vi "_DP2TDMData.vi"(6 "chunk size":u32=10000000, 8 "error in (no error)":errorcluster, 10 "DataPlugin Object in":refnum<k20>, 11 "TDM Object in":refnum<k20>) -> (0 "error out":errorcluster, 2 "DataPlugin object out":refnum<k20>, 3 "TDM Object out":refnum<k20>)   [LabVIEW 2017]
doc: "Transfers data from the TDM storage to the TDMS file in chunks of a size specified in samples until all samples have been transferred."
uses:
  <vilib>/Utility/tdmsutil.llb/TDM2TDMSDatatypes.ctl
  <vilib>/Platform/storage/lvStorage.llb/_saveStringChannel.vi
  <vilib>/Platform/storage/lvStorage.llb/_saveInt16Channel.vi
  <vilib>/Platform/storage/lvStorage.llb/_saveFloat32Channel.vi
  <vilib>/Platform/storage/lvStorage.llb/_saveUInt8Channel.vi
  <vilib>/Platform/storage/lvStorage.llb/_saveInt32Channel.vi
  <vilib>/Platform/storage/lvStorage.llb/_saveFloat64Channel.vi
  <vilib>/Platform/storage/lvStorage.llb/_saveDateTimeChannel.vi
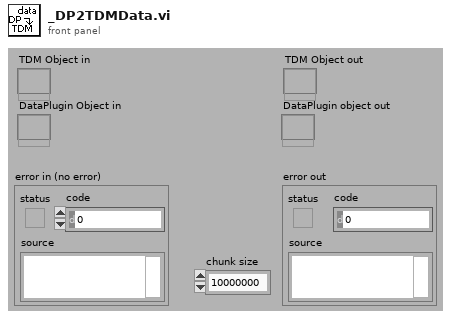
[diagram p1: front panel]
types:
  T1 = typedef "TDM2TDMSDatatypes.ctl" = enum16{"DT_UNKNOWN", "DT_STRING", "DT_SHORT", "DT_FLOAT", "DT_BOOLEAN", "DT_BYTE", "DT_LONG", "DT_DOUBLE", "DT_LONGLONG", "DT_ID", "DT_DATE", "DT_BYTESTR", "DT_BLOB", "DT_COMPLEX", "DT_DCOMPLEX", "DT_ENUM"}
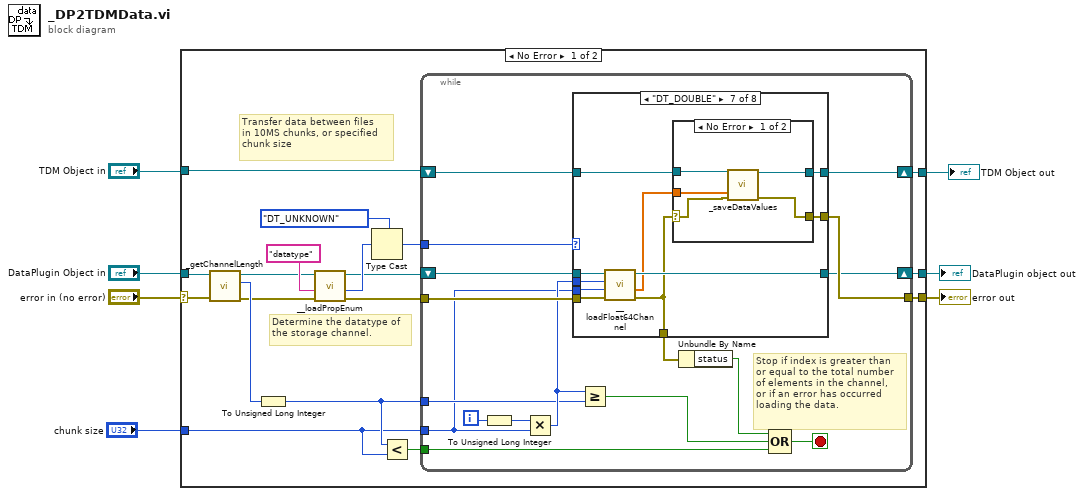
[diagram p0: block diagram]
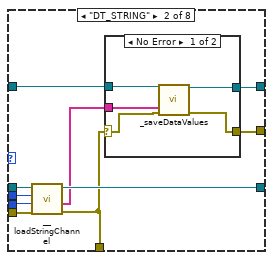
[diagram p3: hidden frame]
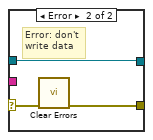
[diagram p4: hidden frame]
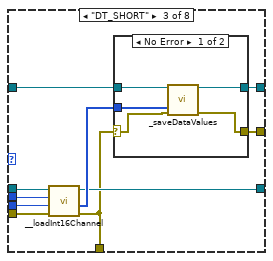
[diagram p5: hidden frame]
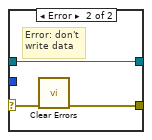
[diagram p6: hidden frame]
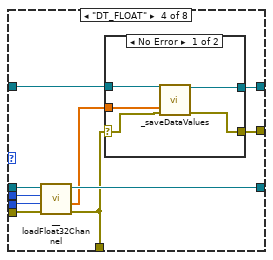
[diagram p7: hidden frame]
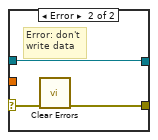
[diagram p8: hidden frame]
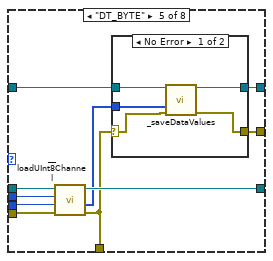
[diagram p9: hidden frame]
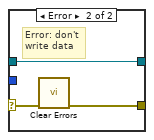
[diagram p10: hidden frame]
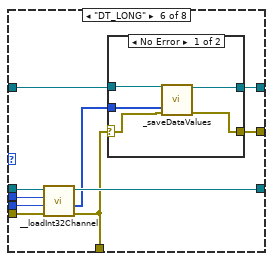
[diagram p11: hidden frame]
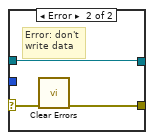
[diagram p12: hidden frame]
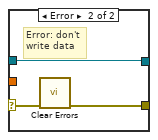
[diagram p13: hidden frame]
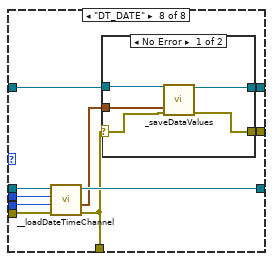
[diagram p14: hidden frame]
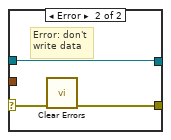
[diagram p15: hidden frame]
diagram:
  n1 = case shown="No Error" "error in (no error)" {
    selector: "error in (no error)" -> [w20 w172]
    tunnel: [w24 w174] -> w1
    tunnel: "DataPlugin Object in" -> [w21 w173]
    tunnel: "TDM Object in" -> [w23 w174]
    tunnel: [w22 w173] -> w2
    tunnel: [w25 w172] -> w7
    tunnel: "chunk size" -> [w9 _]
    frame No Error {
      # "Determine the datatype of\nthe storage channel."
      # "Transfer data between files\nin 10MS chunks, or specified\nchunk size"
      n2 = call <vilib>:"_getChannelLength.vi"("error in (no error)"=w20, "channel refnum in"=w21) -> ("error out"=w14:errorcluster, "channel length"=w19:i32, "channel refnum out"=w15:refnum<k20>)  [unwired: 3 in]
      n3 = To Unsigned Long Integer(number=w19) -> (unsigned 32bit integer=w10:u32)
      n4 = call <vilib>:"__loadPropEnum.vi"("error in (no error)"=w14, "Property name"="datatype", "storage refnum"=w15) -> ("error out"=w12:errorcluster, "Value"=w16:u16, "dup storage refnum"=w13:refnum<k20>)  [unwired: 5 in, 1 out]
      n5 = Type Cast(type=TDM2TDMSDatatypes."DT_UNKNOWN" ("Data type"), x=w16) -> (*(type *) &x=w11:T1)
      n6 = Less?(x=w10, y=w9) -> (x < y?=w8:bool)
      n7 = while {
        shift-right: [w42] -> w24
        shift-left: w23 -> [w40]
        shift-right: [w31] -> w22
        shift-left: w13 -> [w34]
        tunnel: [w39] -> w25
        tunnel: w10 -> [w28]
        tunnel: w9 -> [w27]
        tunnel: w12 -> [w35]
        tunnel: w11 -> [w36]
        tunnel: w8 -> [w26]
        i -> [w38]
        stop <- w41 stop-if-true
        # "Stop if index is greater than\nor equal to the total number\nof elements in the channel,\nor if an error has occurred\nloading the data."
        n8 = To Unsigned Long Integer(number=w38) -> (unsigned 32bit integer=w37:u32)
        n9 = Multiply(x=w37, y=w27) -> (x*y=w32:u32)
        n10 = case shown="\"DT_DOUBLE\"" w36 {
          tunnel: [w45 w50 w64 w86 w104 w121 w140 w157] -> w42
          tunnel: w40 -> [w45 w46 w73 w82 w103 w120 w138 w156]
          tunnel: [w44 w49 w66 w85 w100 w122 w139 w158] -> w39
          tunnel: w35 -> [w44 w54 w71 w90 w108 w126 w144 w162]
          tunnel: w34 -> [w43 w55 w72 w91 w109 w127 w145 w163]
          tunnel: w32 -> [_ w53 w70 w89 w107 w124 w143 w161]
          tunnel: w27 -> [_ w52 w69 w88 w106 w123 w142 w160]
          tunnel: [w43 w51 w67 w87 w105 w125 w141 w159] -> w31
          tunnel: [w44 w48 w65 w84 w102 w118 w136 w154] -> w30
          frame "DT_UNKNOWN", Default {
          }
          frame "DT_STRING" {
            n11 = call <vilib>:"__loadStringChannel.vi"("error in (no error)"=w54, "Count"=w52, "Index"=w53, "Data object in"=w55) -> ("error out"=w48:errorcluster, "Values"=w47:string[], "Data object out"=w51:refnum<k20>)  [unwired: 1 out]
            n12 = case shown="No Error" w48 {
              tunnel: [w60 w62] -> w49
              selector: w48 -> [w59 w63]
              tunnel: [w58 w61] -> w50
              tunnel: w47 -> [w57 _]
              tunnel: w46 -> [w56 w61]
              frame No Error {
                n13 = call-poly <vilib>:"_saveDataValues.vi"("Data object in"=w56, "Values"=w57, "error in (no error)"=w59) -> ("Data object out"=w58:refnum<k20>, "error out"=w60:errorcluster)  [unwired: 10 in, 1 out]
              }
              frame Error {
                # "Error: don't\nwrite data"
                n14 = call <vilib>:"Clear Errors.vi"("error in (no error)"=w63) -> ("error out"=w62:errorcluster)  [unwired: 5 in, 1 out]
              }
            }
          }
          frame "DT_SHORT" {
            n15 = call <vilib>:"__loadInt16Channel.vi"("error in (no error)"=w71, "Count"=w69, "Index"=w70, "Data object in"=w72) -> ("error out"=w65:errorcluster, "Values"=w68:i16[], "Data object out"=w67:refnum<k20>)  [unwired: 1 out]
            n16 = case shown="No Error" w65 {
              tunnel: w73 -> [w78 w79]
              tunnel: [w76 w80] -> w66
              selector: w65 -> [w75 w81]
              tunnel: w68 -> [w74 _]
              tunnel: [w77 w79] -> w64
              frame No Error {
                n17 = call-poly <vilib>:"_saveDataValues.vi"("Data object in"=w78, "Values"=w74, "error in (no error)"=w75) -> ("Data object out"=w77:refnum<k20>, "error out"=w76:errorcluster)  [unwired: 10 in, 1 out]
              }
              frame Error {
                # "Error: don't\nwrite data"
                n18 = call <vilib>:"Clear Errors.vi"("error in (no error)"=w81) -> ("error out"=w80:errorcluster)  [unwired: 5 in, 1 out]
              }
            }
          }
          frame "DT_FLOAT" {
            n19 = call <vilib>:"__loadFloat32Channel.vi"("error in (no error)"=w90, "Count"=w88, "Index"=w89, "Data object in"=w91) -> ("error out"=w84:errorcluster, "Values"=w83:sgl[], "Data object out"=w87:refnum<k20>)  [unwired: 1 in]
            n20 = case shown="No Error" w84 {
              tunnel: [w95 w98] -> w85
              selector: w84 -> [w94 w99]
              tunnel: w83 -> [w93 _]
              tunnel: [w96 w97] -> w86
              tunnel: w82 -> [w92 w97]
              frame No Error {
                n21 = call-poly <vilib>:"_saveDataValues.vi"("Data object in"=w92, "Values"=w93, "error in (no error)"=w94) -> ("Data object out"=w96:refnum<k20>, "error out"=w95:errorcluster)  [unwired: 10 in, 1 out]
              }
              frame Error {
                # "Error: don't\nwrite data"
                n22 = call <vilib>:"Clear Errors.vi"("error in (no error)"=w99) -> ("error out"=w98:errorcluster)  [unwired: 5 in, 1 out]
              }
            }
          }
          frame "DT_BYTE" {
            n23 = call <vilib>:"__loadUInt8Channel.vi"("error in (no error)"=w108, "Count"=w106, "Index"=w107, "Data object in"=w109) -> ("error out"=w102:errorcluster, "Values"=w101:u8[], "Data object out"=w105:refnum<k20>)  [unwired: 1 out]
            n24 = case shown="No Error" w102 {
              tunnel: [w113 w116] -> w100
              selector: w102 -> [w112 w117]
              tunnel: [w114 w115] -> w104
              tunnel: w103 -> [w111 w115]
              tunnel: w101 -> [w110 _]
              frame No Error {
                n25 = call-poly <vilib>:"_saveDataValues.vi"("Data object in"=w111, "Values"=w110, "error in (no error)"=w112) -> ("Data object out"=w114:refnum<k20>, "error out"=w113:errorcluster)  [unwired: 10 in, 1 out]
              }
              frame Error {
                # "Error: don't\nwrite data"
                n26 = call <vilib>:"Clear Errors.vi"("error in (no error)"=w117) -> ("error out"=w116:errorcluster)  [unwired: 5 in, 1 out]
              }
            }
          }
          frame "DT_LONG" {
            n27 = call <vilib>:"__loadInt32Channel.vi"("error in (no error)"=w126, "Count"=w123, "Index"=w124, "Data object in"=w127) -> ("error out"=w118:errorcluster, "Values"=w119:i32[], "Data object out"=w125:refnum<k20>)  [unwired: 1 out]
            n28 = case shown="No Error" w118 {
              tunnel: [w131 w134] -> w122
              selector: w118 -> [w130 w135]
              tunnel: w119 -> [w129 _]
              tunnel: [w132 w133] -> w121
              tunnel: w120 -> [w128 w133]
              frame No Error {
                n29 = call-poly <vilib>:"_saveDataValues.vi"("Data object in"=w128, "Values"=w129, "error in (no error)"=w130) -> ("Data object out"=w132:refnum<k20>, "error out"=w131:errorcluster)  [unwired: 10 in, 1 out]
              }
              frame Error {
                # "Error: don't\nwrite data"
                n30 = call <vilib>:"Clear Errors.vi"("error in (no error)"=w135) -> ("error out"=w134:errorcluster)  [unwired: 5 in, 1 out]
              }
            }
          }
          frame "DT_DOUBLE" {
            n31 = call <vilib>:"__loadFloat64Channel.vi"("error in (no error)"=w144, "Count"=w142, "Index"=w143, "Data object in"=w145) -> ("error out"=w136:errorcluster, "Values"=w137:dbl[], "Data object out"=w141:refnum<k20>)  [unwired: 1 out]
            n32 = case shown="No Error" w136 {
              tunnel: [w149 w152] -> w139
              selector: w136 -> [w148 w153]
              tunnel: w137 -> [w147 _]
              tunnel: [w150 w151] -> w140
              tunnel: w138 -> [w146 w151]
              frame No Error {
                n33 = call-poly <vilib>:"_saveDataValues.vi"("Data object in"=w146, "Values"=w147, "error in (no error)"=w148) -> ("Data object out"=w150:refnum<k20>, "error out"=w149:errorcluster)  [unwired: 10 in, 1 out]
              }
              frame Error {
                # "Error: don't\nwrite data"
                n34 = call <vilib>:"Clear Errors.vi"("error in (no error)"=w153) -> ("error out"=w152:errorcluster)  [unwired: 5 in, 1 out]
              }
            }
          }
          frame "DT_DATE" {
            n35 = call <vilib>:"__loadDateTimeChannel.vi"("error in (no error)"=w162, "Count"=w160, "Index"=w161, "Data object in"=w163) -> ("error out"=w154:errorcluster, "Values"=w155:timestamp[], "Data object out"=w159:refnum<k20>)  [unwired: 1 out]
            n36 = case shown="No Error" w154 {
              tunnel: [w167 w170] -> w158
              selector: w154 -> [w166 w171]
              tunnel: w155 -> [w165 _]
              tunnel: [w168 w169] -> w157
              tunnel: w156 -> [w164 w169]
              frame No Error {
                n37 = call-poly <vilib>:"_saveDataValues.vi"("Data object in"=w164, "Values"=w165, "error in (no error)"=w166) -> ("Data object out"=w168:refnum<k20>, "error out"=w167:errorcluster)  [unwired: 10 in, 1 out]
              }
              frame Error {
                # "Error: don't\nwrite data"
                n38 = call <vilib>:"Clear Errors.vi"("error in (no error)"=w171) -> ("error out"=w170:errorcluster)  [unwired: 5 in, 1 out]
              }
            }
          }
        }
        n39 = Greater Or Equal?(x=w32, y=w28) -> (x >= y?=w29:bool)
        n40 = Unbundle By Name(w30) -> ("status"=w33:bool)
        n41 = Compound Arithmetic op=OR(w33, w29, w26) -> (w41:bool)
      }
    }
    frame Error {
    }
  }
  "error out" <- w7
  "DataPlugin object out" <- w2
  "TDM Object out" <- w1
